vi "DataDrag2.vi"(0 "XRef":T10, 1 "Point":T8, 2 "String":T5, 3 "Path":T7, 4 "ProjectRef":T6, 5 "State In":T1) -> (14 "Reply":T4, 15 "State Out":T1)   [LabVIEW 2015, in "Async-And-Forget.xnode"]
doc: "This ability VI is called by LabVIEW when your XNode receives a data drag. Some combination of String, Path, and ProjectRef will have a non-empty value depending what data the drag element can supply and what data CanAcceptDataDrag2 indicated your XNode could receive. Currently Point is always (0, 0). Use Reply to inform LabVIEW of any actions it needs to take.\n\nDefault behavior: None.\n\nThis ability provides UI and OS messages are handled.\n\nSee also: CanAcceptDataDrag2, GetDataForDrag"
uses:
  Async-And-Forget.xnode
  <vilib>/XNodeSupport/XNodeXNodeRef.ctl
  <vilib>/XNodeSupport/XNodePoint.ctl
  <vilib>/XNodeSupport/XNodeInt.ctl
  <vilib>/XNodeSupport/XNodeString.ctl
  <vilib>/XNodeSupport/XNodePath.ctl
  <vilib>/XNodeSupport/XNodeProjectRef.ctl
  State.ctl
  <vilib>/Utility/miscctls.llb/LVRectTypeDef.ctl
  <vilib>/picture/picture.llb/imagedata.ctl
  <vilib>/XNodeSupport/XNodeStringArray.ctl
  <vilib>/XNodeSupport/NI_XNodeSupport.lvlib
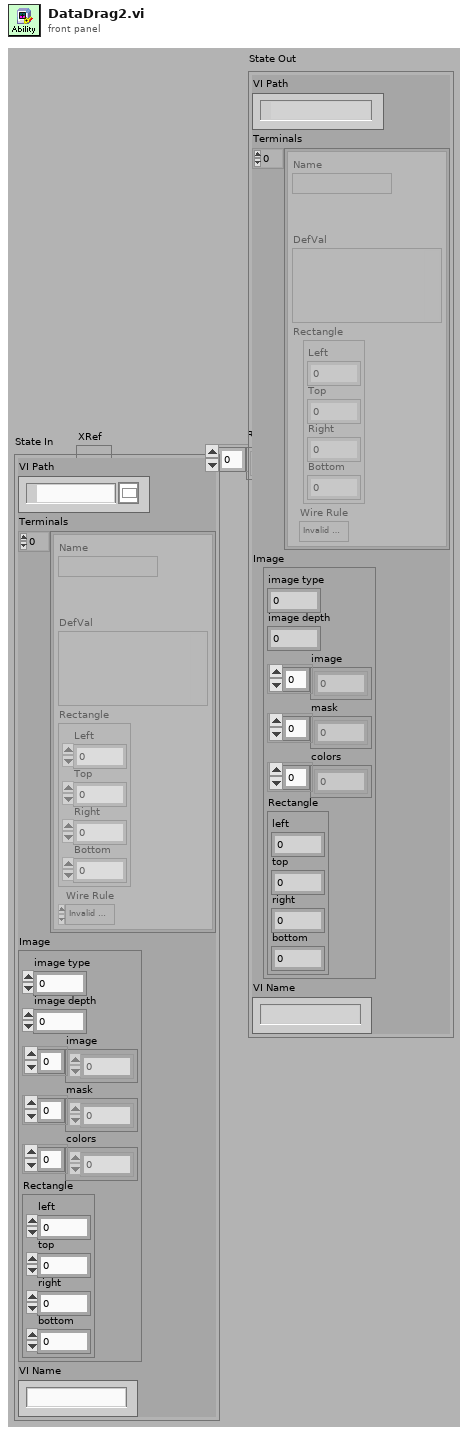
[diagram p1: front panel]
types:
  T1 = typedef "Async-And-Forget.xnode/State.ctl" = cluster{"VI Path":path, "Terminals":cluster{"Name":string, "DefVal":variant, "Rectangle":T2, "Wire Rule":enum16{"Invalid Wire Rule", "Required", "Recommended", "Optional", "Dynamic Dispatch"}}[], "Image":T3, "VI Name":string}
  T2 = typedef "LVRectTypeDef.ctl" = cluster{"Left":i16, "Top":i16, "Right":i16, "Bottom":i16}
  T3 = typedef "imagedata.ctl" = cluster{"image type":i32, "image depth":i32, "image":u8[], "mask":u8[], "colors":u32[], "Rectangle":cluster{"left":i16, "top":i16, "right":i16, "bottom":i16}}
  T4 = typedef "NI_XNodeSupport.lvlib/XNodeStringArray.ctl" = T5[]
  T5 = typedef "NI_XNodeSupport.lvlib/XNodeString.ctl" = string
  T6 = typedef "NI_XNodeSupport.lvlib/XNodeProjectRef.ctl" = refnum<vi>
  T7 = typedef "NI_XNodeSupport.lvlib/XNodePath.ctl" = path
  T8 = typedef "NI_XNodeSupport.lvlib/XNodePoint.ctl" = cluster{"H":T9, "V":T9}
  T9 = typedef "NI_XNodeSupport.lvlib/XNodeInt.ctl" = i32
  T10 = typedef "NI_XNodeSupport.lvlib/XNodeXNodeRef.ctl" = refnum<vi>
  T11 = enum16{"Invalid Wire Rule", "Required", "Recommended", "Optional", "Dynamic Dispatch"}[]
  T12 = cluster{"Label.Text":string, "DefVal":variant, "Rectangle":T2, "Wire Rule":enum16{"Invalid Wire Rule", "Required", "Recommended", "Optional", "Dynamic Dispatch"}}[]
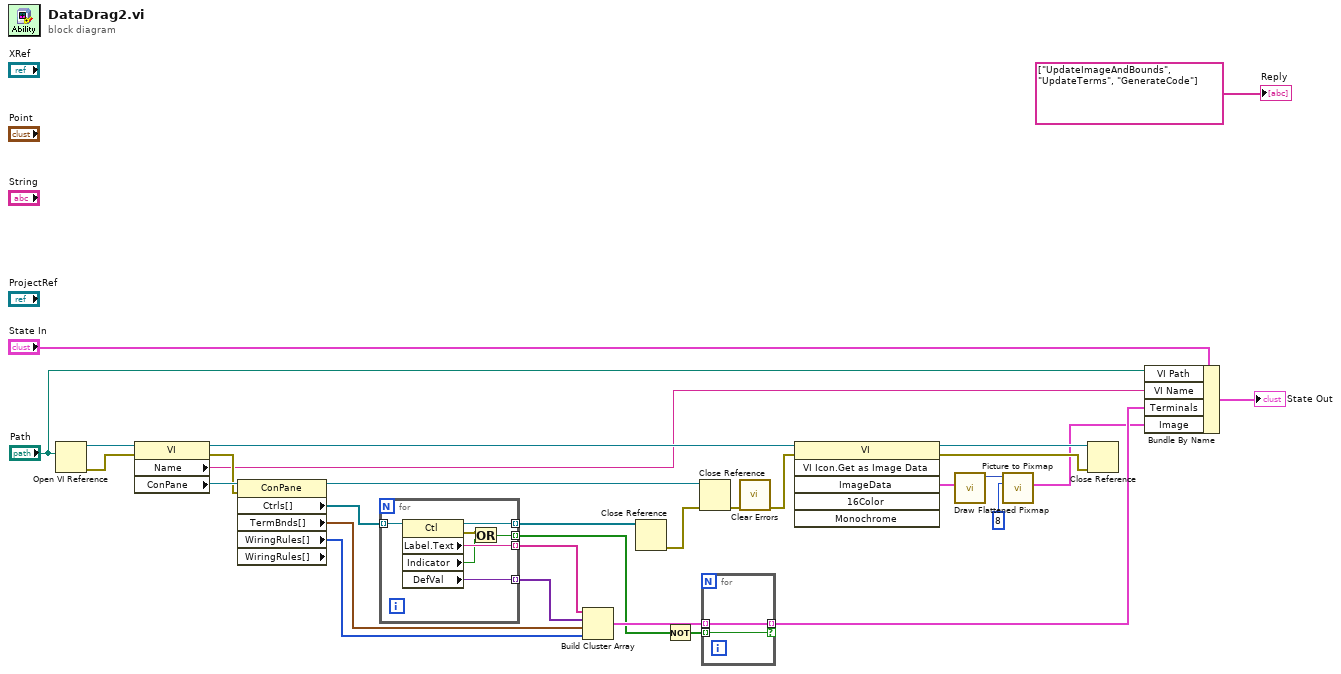
[diagram p0: block diagram]
diagram:
  n1 = Open VI Reference(vi path="Path") -> (vi reference=w30:refnum<vi>, error out=w11:errorcluster)  [unwired: 5 in]
  n2 = property class="VI"(reference=w30, error in=w11) -> (reference out=w18:refnum<vi>, error out=w23:errorcluster, "Name"=w10:string, "ConPane"=w29:refnum<vi>)
  n3 = property class="ConPane" props=["Ctrls[]", "TermBnds[]", "WiringRules[]", "WiringRules[]"](reference=w29, error in=w23) -> (reference out=w12:refnum<vi>, "Ctrls[]"=w28:refnum<vi>[], "TermBnds[]"=w26:T2[], "WiringRules[]"=w27:T11)  [unwired: 2 out]
  n4 = for {
    tunnel: w28 -> [w37] mode=indexing
    tunnel: [w36] -> w24 mode=indexing
    tunnel: [w35] -> w25 mode=indexing
    tunnel: [w34] -> w22 mode=indexing
    tunnel: [w31] -> w7 mode=indexing
    n5 = property class="Ctl"(reference=w37) -> (reference out=w34:refnum<vi>, error out=w33:errorcluster, "Label.Text"=w36:string, "Indicator"=w32:bool, "DefVal"=w35:variant)  [unwired: 1 in]
    n6 = Or(x=w33, y=w32) -> (x .or. y?=w31:bool)
  }
  n7 = Build Cluster Array(w24, w25, w26, w27) -> (w9:T12)
  n8 = Close Reference(reference=w22) -> (error out=w21:errorcluster)  [unwired: 1 in]
  n9 = Not(x=w7) -> (.not. x?=w6:bool[])
  n10 = Close Reference(reference=w12, error in (no error)=w21) -> (error out=w17:errorcluster)
  n11 = for {
    tunnel: w9 -> [w39] mode=indexing
    tunnel: [w39] -> w8 mode=indexing if=w38
    tunnel: w6 -> [w38] mode=indexing
  }
  n12 = call <vilib>:"Clear Errors.vi"("error in (no error)"=w17) -> ("error out"=w13:errorcluster)  [unwired: 5 in, 1 out]
  n13 = invoke class="VI" method="VI Icon.Get as Image Data"(reference=w18, error in=w13) -> (reference out=w16:refnum<vi>, error out=w15:errorcluster, "ImageData"=w4:T3)  [unwired: 4 in, 3 out]
  n14 = call <vilib>:"Draw Flattened Pixmap.vi"("image data"=w4) -> ("new picture"=w3:picture)  [unwired: 8 in]
  n15 = call <vilib>:"Picture to Pixmap.vi"("depth"=8, "picture"=w3) -> ("image data"=w1:T3)  [unwired: 8 in, 1 out]
  n16 = Close Reference(reference=w16, error in (no error)=w15) -> ()  [unwired: 1 out]
  n17 = Bundle By Name(cluster="State In", "VI Path"="Path", "VI Name"=w10, "Terminals"=w8, "Image"=w1) -> (→"State Out":T1)
  "Reply" <- string[] ["UpdateImageAndBounds", "UpdateTerms", "GenerateCode"] ("Reply")
